vi "Create Class Folder.vi"(11 "Actor Script Strategy in":refnum<class "Actor Script Strategy.lvclass">) -> (3 "Actor Script Strategy out":refnum<class "Actor Script Strategy.lvclass">)   [LabVIEW 2021, in "_Create From Template.lvlib" / "Script Strategy.lvlib" / "Actor Script Strategy.lvclass"]
uses:
  Actor Script Strategy.lvclass
  Actor Script Strategy.lvclass/Actor Script Strategy.ctl
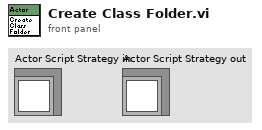
[diagram p1: front panel]
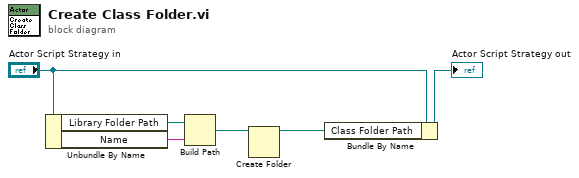
[diagram p0: block diagram]
diagram:
  n1 = Unbundle By Name("Actor Script Strategy in") -> ("Library Folder Path"=w5:path, "Name"=w1:string)
  n2 = Build Path(base path=w5, name or relative path=w1) -> (appended path=w4:path)
  n3 = Create Folder(path (use dialog)=w4) -> (created path=w2:path)  [unwired: 2 in, 2 out]
  n4 = Bundle By Name(cluster="Actor Script Strategy in", "Class Folder Path"=w2) -> (→"Actor Script Strategy out":refnum<class "Actor Script Strategy.lvclass">)
